vi "Generate Report.vi"(8 "error in (no error)":errorcluster, 11 "Network Test in":refnum<class "Network Test.lvclass">) -> (0 "error out":errorcluster, 3 "Network Test out":refnum<class "Network Test.lvclass">)   [LabVIEW 2017, in "Network Test.lvlib" / "Network Test.lvclass"]
uses:
  Network Test.lvclass
  Network Test.lvclass/Network Test.ctl
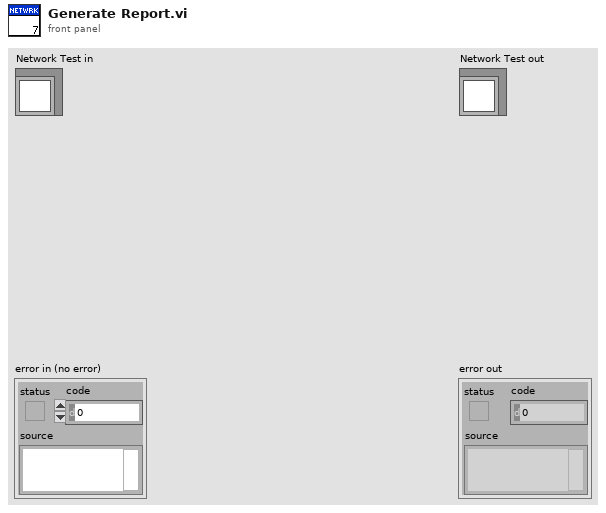
[diagram p1: front panel]
types:
  T1 = typedef "Paths.ctl" = cluster{"Data Directory":path, "Test Config Dir":path, "Error Logs":path, "Event Logs":path, "Settings.Json":path, "Reports Directory":path}
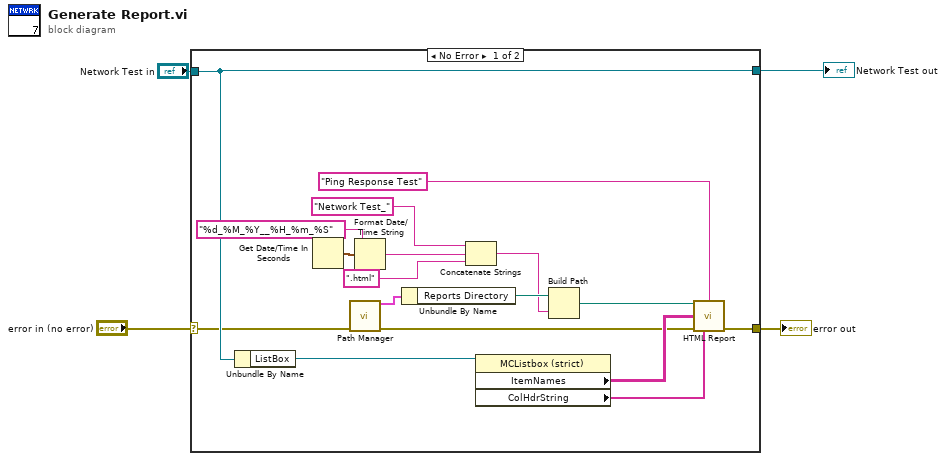
[diagram p0: block diagram]
diagram:
  n1 = case shown="No Error" "error in (no error)" {
    selector: "error in (no error)" -> [w8 w22]
    tunnel: [w10 w22] -> w4
    tunnel: "Network Test in" -> [w9 w23]
    tunnel: [w9 w23] -> w1
    frame No Error {
      n2 = Unbundle By Name(w9) -> ("ListBox"=w15:refnum<vi>)
      n3 = Get Date/Time In Seconds() -> (seconds since 1Jan1904=w7:timestamp)
      n4 = call "Path Manager.vi"("Error in (no error)"=w8) -> ("Cluster"=w21:T1, "Error out"=w11:errorcluster)  [unwired: 13 in]
      n5 = Format Date/Time String(time format string (%c)="%d_%M_%Y__%H_%m_%S", seconds (now)=w7) -> (date/time string=w5:string)  [unwired: 1 in]
      n6 = Unbundle By Name(w21) -> ("Reports Directory"=w19:path)
      n7 = Concatenate Strings("Network Test_", w5, ".html" ("string")) -> (w18:string)
      n8 = property class="MCListbox (strict)"(reference=w15) -> ("ItemNames"=w14:string[][], "ColHdrString"=w13:string[])  [unwired: 1 in, 2 out]
      n9 = Build Path(base path=w19, name or relative path=w18) -> (appended path=w17:path)
      n10 = call "HTML Report.vi"("report file path"=w17, "Column Headers"=w13, "Header"="Ping Response Test", "Table Data"=w14, "error in (no error)"=w11) -> ("error out"=w10:errorcluster)  [unwired: 10 in]
    }
    frame Error {
    }
  }
  "error out" <- w4
  "Network Test out" <- w1
